vi "Test Numeric Upper Compare GELE in Report.vi"(11 "Test Case In":refnum<class "Report CSV Content Test.lvclass">) -> (0 "error out":errorcluster, 3 "Test Case Out":refnum<class "Report CSV Content Test.lvclass">)   [LabVIEW 2020, in "Report CSV Content Test.lvclass"]
uses:
  Report CSV Content Test.lvclass
  4993e8ee-a06a-463a-9684-69129f64d5ce.vi
  source/Test Result Handler/TestStand Result Handler.lvclass
  Mock Configuration/Mock Configuration.lvclass
  <vilib>/Astemes/LMock/LMock.lvlib
  <vilib>/Astemes/LMock/One Identical Inputs.vi
  <vilib>/Astemes/LMock/LMock One.lvlib
  <vilib>/Astemes/LMock/LMock Verifier.lvclass
  C:/Program Files (x86)/National Instruments/LabVIEW 2020/vi.lib/Astemes/LMock/Mock.lvclass
  C:/git/astemes-excel-report-teststand-plugin/tests/Mock Configuration/Mock Configuration.lvclass
  C:/git/astemes-excel-report-teststand-plugin/source/Astemes_CSVReportGenerator/Configuration/Configuration.lvclass
  C:/Program Files (x86)/National Instruments/LabVIEW 2020/vi.lib/Astemes/LUnit/Test Case.lvclass
  C:/Program Files (x86)/National Instruments/LabVIEW 2020/vi.lib/Astemes/LUnit/LUnit Runnable.lvclass
  C:/git/astemes-excel-report-teststand-plugin/tests/Test Report CSV Content/Report CSV Content Test.lvclass
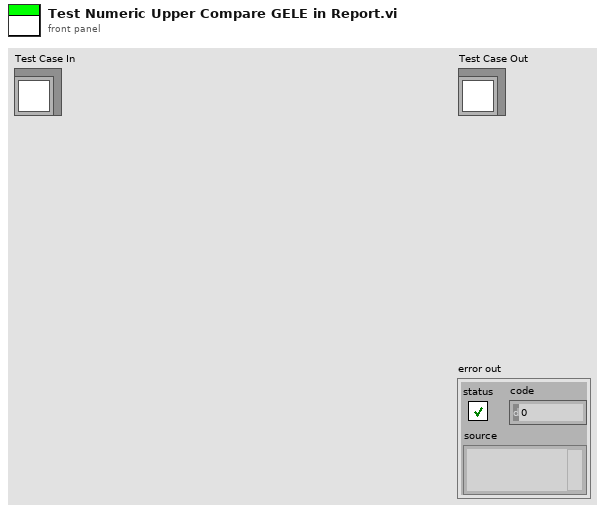
[diagram p1: front panel]
types:
  T1 = typedef "Astemes_CSVReportPlugin.lvlib/TestStand Result Handler.lvclass/TestStand Result.ctl" = cluster{"error in (no error)":errorcluster, "ReportText":string, "TS":cluster{"Index":i32, "BlockLevel":i32, "StartTime":dbl, "Id":i32, "StepType":string, "StepID":string, "StepGroup":string, "StepName":string}, "Status":string}
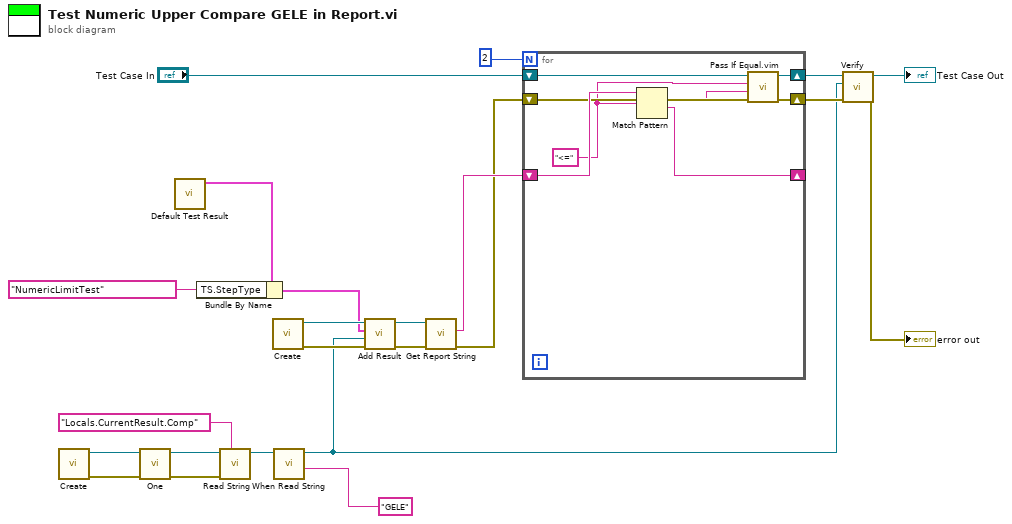
[diagram p0: block diagram]
diagram:
  n1 = call "Create.vi"() -> ("error out"=w12:errorcluster, "Mock Class Generator out"=w11:refnum<class "Mock Configuration.lvclass">)  [unwired: 10 in]
  n2 = call-poly <vilib>:"One.vi"("error in (no error)"=w12, "Mock in"=w11) -> ("error out"=w9:errorcluster, "Mock out"=w10:refnum<class "Mock Configuration.lvclass">)  [unwired: 8 in]
  n3 = call "Default Test Result.vi"() -> ("TestStand Result"=w17:T1)  [unwired: 11 in]
  n4 = Bundle By Name(cluster=w17, "TS.StepType"="NumericLimitTest" ("Status")) -> (w16:T1)
  n5 = call-dynamic "Read String.vi"("key"="Locals.CurrentResult.Comp", "error in (no error)"=w9, "Configuration In"=w10) -> ("Configuration Out"=w8:refnum<class "Mock Configuration.lvclass">)  [unwired: 6 in, 2 out]
  n6 = call "Create.vi"() -> ("error out"=w20:errorcluster, "Test Result Handler"=w21:refnum<class "TestStand Result Handler.lvclass">)  [unwired: 10 in]
  n7 = call "When Read String.vi"("value"="GELE", "Configuration In"=w8) -> ("Configuration Out"=w3:refnum<class "Mock Configuration.lvclass">)  [unwired: 9 in]
  n8 = call "Add Result.vi"("error in (no error)"=w20, "Sequenc Context"=w3, "TestStand Result"=w16, "TestStand Result Handler In"=w21) -> ("error out"=w18:errorcluster, "TestStand Result Handler Out"=w19:refnum<class "TestStand Result Handler.lvclass">)  [unwired: 6 in]
  n9 = call "Get Report String.vi"("error in (no error)"=w18, "TestStand Result Handler In"=w19) -> ("error out"=w13:errorcluster, "Report Text"=w15:string)  [unwired: 8 in]
  n10 = for {
    N: 2 -> [_]
    shift-right: [w27] -> w5
    shift-left: "Test Case In" -> [w31]
    shift-right: [w30] -> w22
    shift-left: w13 -> [w28]
    shift-right: [w24] -> _
    shift-left: w15 -> [w29]
    w26 = "<=" ("regular expression")
    n11 = Match Pattern(string=w29, regular expression=w26) -> (match substring=w25:string, after substring=w24:string)  [unwired: 1 in, 2 out]
    n12 = call "Pass If Equal.vim"("error in (no error)"=w28, "Actual"=w25, "Expected"=w26, "LUnit Test Case In"=w31) -> ("error out"=w30:errorcluster, "LUnit Test Case Out"=w27:refnum<class "Report CSV Content Test.lvclass">)  [unwired: 6 in]
  }
  n13 = call <vilib>:"Verify.vi"("error in (no error)"=w22, "Mock"=w3, "LUnit Test Case In"=w5) -> ("error out"=→"error out":errorcluster, "LUnit Test Case Out"=→"Test Case Out":refnum<class "Report CSV Content Test.lvclass">)  [unwired: 7 in]
